vi "Increment.vi"(8 "error in (no error)":errorcluster, 11 "SimpleAF in":refnum<class "Counter.lvclass">) -> (0 "error out":errorcluster, 3 "SimpleAF out":refnum<class "Counter.lvclass">)   [LabVIEW 2013, in "Counter.lvclass"]
uses:
  Counter.lvclass
  Counter.lvclass/Counter.ctl
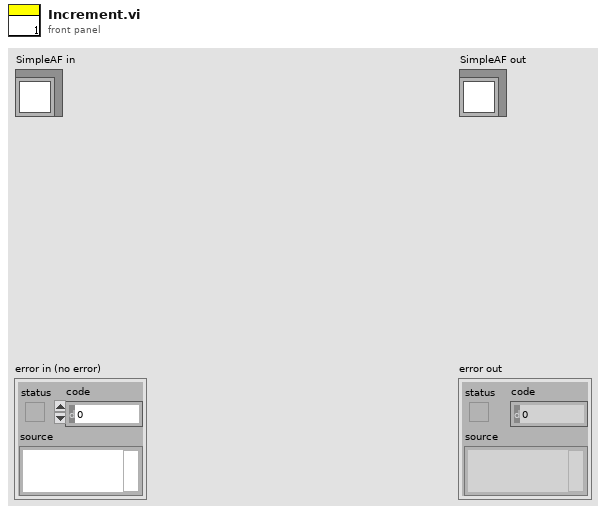
[diagram p1: front panel]
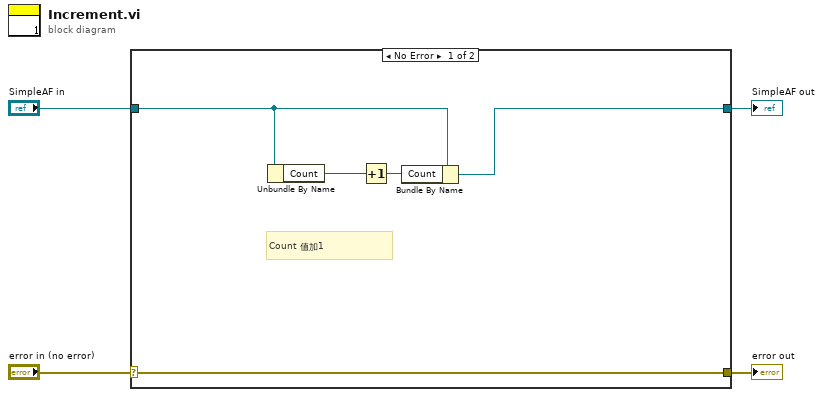
[diagram p0: block diagram]
diagram:
  n1 = case shown="No Error" "error in (no error)" {
    selector: "error in (no error)" -> [w9 w11]
    tunnel: [w9 w11] -> w3
    tunnel: [w5 w10] -> w1
    tunnel: "SimpleAF in" -> [w6 w10]
    frame No Error {
      # "Count 值加1"
      n2 = Unbundle By Name(w6) -> ("Count"=w8:i32)
      n3 = Increment(x=w8) -> (x+1=w7:i32)
      n4 = Bundle By Name(cluster=w6, "Count"=w7) -> (w5:refnum<class "Counter.lvclass">)
    }
    frame Error {
    }
  }
  "error out" <- w3
  "SimpleAF out" <- w1
